vi "Register Process (Default).vi"(8 "error in (no error)":errorcluster, 9 "Process Name (optional)":string, 11 "SMO":refnum<class "SMO.lvclass">) -> (0 "error out":errorcluster, 3 "SelfRef":refnum<class "SMO.lvclass">)   [LabVIEW 2021, in "smo.lvlib" / "SMO.lvclass"]
doc: "Philosophy of Registration of SMOs\n=========================\nOverriding \"Process.vi\" is mandatory (Must Call Parent) to allow the framework to achieve necessary housekeeping functionality.\nThere are two ways the developer can override a process: a) by extending its functionalities (EXTENSION) or b) by overwriting its functionalities (OVERWRITE).\nEven if the parent method has to be called, the framework allows the developer to request that its parent process not run (overwriting).\n\nAt this point, it becomes the responsibility of the parent process to decide if it should comply with this request or ignore it. If it chooses to ignore its child's request,\nthe process will be extended. This is meant to allow a process to do critical functions necessary to its performance even if the child requests to overwrite it.\n\nIn a nutshell, each process can decide at runtime if it allows itself to be overwritten or simply extended by a more specific implementation."
uses:
  SMO.lvclass
  Typedefs/Parent Call--Enum.ctl
  SMO.lvclass/SMO.ctl
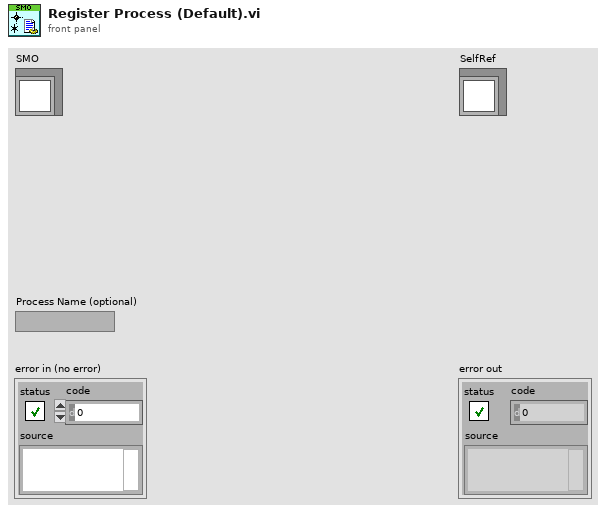
[diagram p1: front panel]
types:
  T1 = typedef "smo.lvlib/SMO.lvclass/Parent Call--Enum.ctl" = enum16{"Allows parent to run", "Does not request parent to run"}
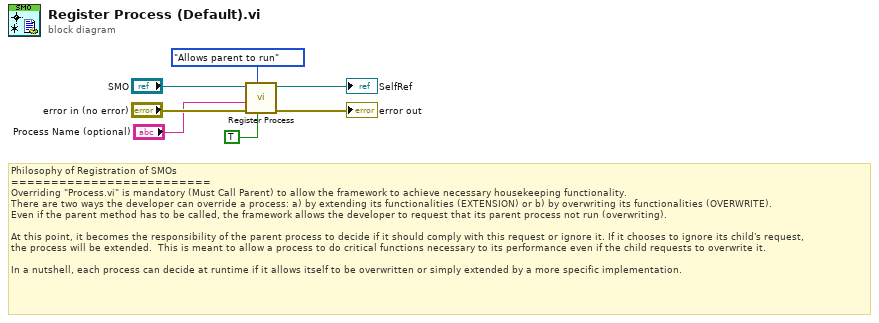
[diagram p0: block diagram]
diagram:
  # "Philosophy of Registration of SMOs\n=========================\nOverriding \"Process.vi\" is mandatory (Must Call Parent) to allow the framework to achieve necessary housekeeping functionality.\nThere are two ways the developer can override a process: a) by extending its functionalities (EXTENSION) or b) by overwriting its functionalities (OVERWRITE).\nEven if the parent method has to be called, the framework allows the developer to request that its parent process not run (overwriting).\n\nAt this point, it becomes the responsibility of the parent process to decide if it should comply with this request or ignore it. If it chooses to ignore its child's request,\nthe process will be extended.  This is meant to allow a process to do critical functions necessary to its performance even if the child requests to overwrite it.\n\nIn a nutshell, each process can decide at runtime if it allows itself to be overwritten or simply extended by a more specific implementation."
  n1 = call "Register Process.vi"("Forces Self to Run (F)"=TRUE, "Parent Call"=Parent_Call--Enum."Allows parent to run", "error in (no error)"="error in (no error)", "Process Name (optional)"="Process Name (optional)", "SMO"="SMO") -> ("error out"=→"error out":errorcluster, "SMO out"=→"SelfRef":refnum<class "SMO.lvclass">)  [unwired: 5 in]
